vi "Main_Processing.vi"(8 "error in":errorcluster, 11 "Queues in":T1) -> (0 "error out":errorcluster)   [LabVIEW 2019]
uses:
  Queue/TypeDef/#TypeDef_MyRIO_Queues.ctl
  TypeDef/#TypeDef_PropFromDAtoDP.ctl
  Communication/TypeDef/#TypeDef_FromPCtoMR.ctl
  Communication/TypeDef/#TypeDef_Command.ctl
  Communication/TypeDef/#TypeDef_ErrorHandler_prop.ctl
  Communication/TypeDef/#TypeDef_FromMRtoPC.ctl
  Communication/TypeDef/#TypeDef_PropGraph.ctl
  Communication/TypeDef/#TypeDef_PropertiesToSave.ctl
  TypeDef/#TypeDef_EnumOp_DataProcessing.ctl
  Communication/TypeDef/#TypeDef_SetGet.ctl
  TypeDef/#TypeDef_MomentValues.ctl
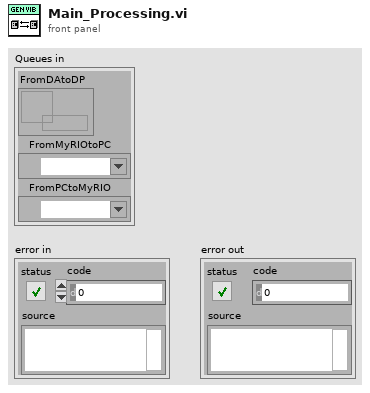
[diagram p1: front panel]
types:
  T1 = typedef "#TypeDef_MyRIO_Queues.ctl" = cluster{"FromDAtoDP":refnum<queue>, "FromMyRIOtoPC":refnum<k21>, "FromPCtoMyRIO":refnum<k21>}
  T2 = typedef "#TypeDef_PropFromDAtoDP.ctl" = cluster{"Accessibility":T3, "RawData":dbl[][], "Counter":i32, "Fs":dbl}
  T3 = typedef "#TypeDef_FromPCtoMR.ctl" = cluster{"Command":T4, "Error?":bool, "Stop":bool, "StopPomiar":bool, "Name":string, "FilesPath":path, "ErrorHandler":T5, "Fs":dbl}
  T4 = typedef "#TypeDef_Command.ctl" = enum16{"Start", "End"}
  T5 = typedef "#TypeDef_ErrorHandler_prop.ctl" = cluster{"Threads":enum16{"Acquisistion", "Data Operation", "Save File"}, "ClearError":bool, "Error Out ":errorcluster, "Error":bool}
  T6 = typedef "#TypeDef_EnumOp_DataProcessing.ctl" = enum16{"Idle", "Init", "Operations", "End", "Error_Shutdown", "ClearError"}
  T7 = typedef "#TypeDef_SetGet.ctl" = enum16{"Set", "Get"}
  T8 = typedef "#TypeDef_MomentValues.ctl" = cluster{"Max":dbl[], "Min":dbl[], "RMS":dbl[], "Init?":bool}
  T9 = typedef "#TypeDef_FromMRtoPC.ctl" = cluster{"Accessibility":T3, "PropGraph":T10, "No Data?":bool, "WaveformData":waveform(dbl)[]}
  T10 = typedef "#TypeDef_PropGraph.ctl" = cluster{"Raw Data":dbl[][], "Poperties":T11, "Power Spectrum / PSD":cluster{"f0":dbl, "df":dbl, "magnitude":dbl[]}[]}
  T11 = typedef "#TypeDef_PropertiesToSave.ctl" = cluster{"RMS values":dbl[], "Max":dbl[], "Min":dbl[], "A(8)":dbl[], "t":dbl, "A(8) Axis":dbl, "Aw":dbl[], "Ak 30min":dbl, "Ak_axis":i32, "Spec":cluster{"f0":dbl, "df":dbl, "magnitude":dbl[]}[]}
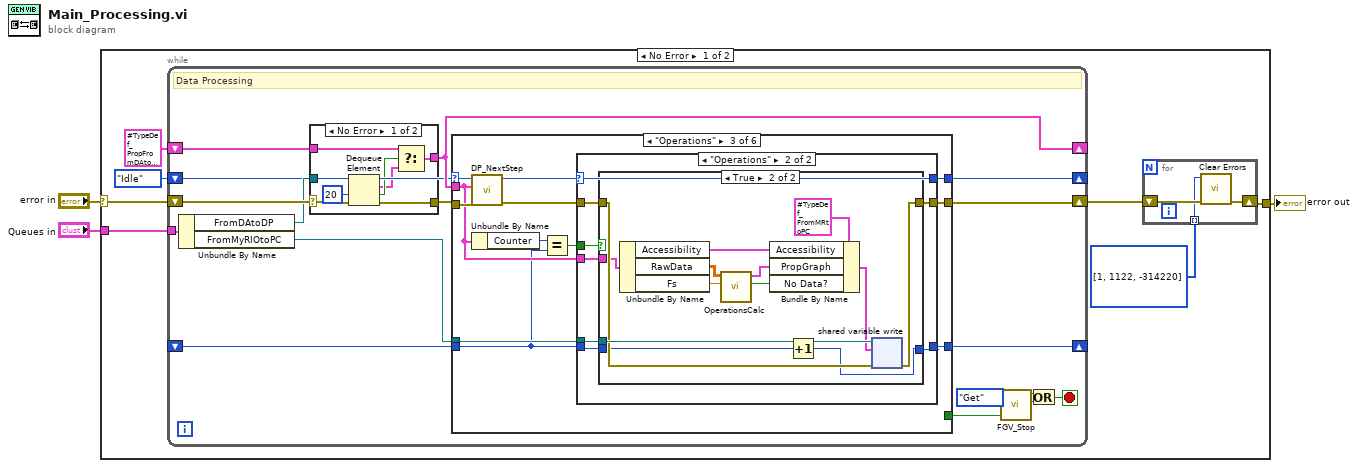
[diagram p0: block diagram]
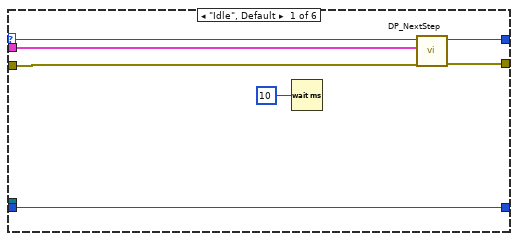
[diagram p3: hidden frame]
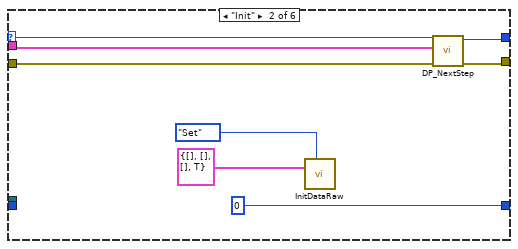
[diagram p4: hidden frame]
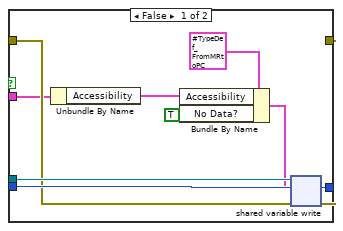
[diagram p6: hidden frame]
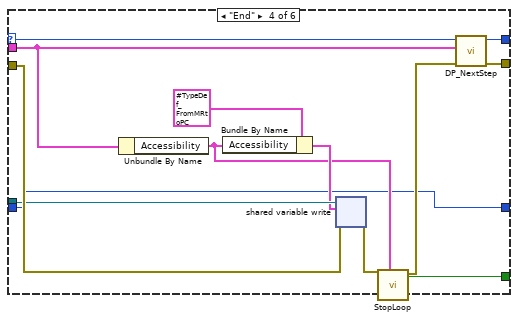
[diagram p7: hidden frame]
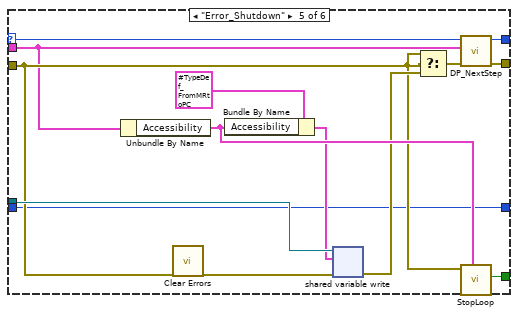
[diagram p8: hidden frame]
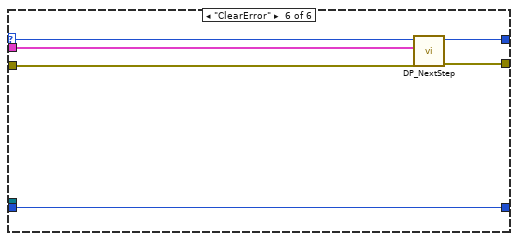
[diagram p9: hidden frame]
diagram:
  n1 = case shown="No Error" "error in" {
    selector: "error in" -> [w10 w133]
    tunnel: "Queues in" -> [w9 _]
    tunnel: [w4 w133] -> w2
    frame No Error {
      n2 = while {
        tunnel: w9 -> [w27]
        shift-right: [w24] -> _
        shift-left: #TypeDef_EnumOp_DataProcessing."Idle" ("EnumOp_DataAcquisition") -> [w21]
        shift-right: [w25] -> w5
        shift-left: w10 -> [w29]
        shift-right: [w22] -> _
        shift-left: T2 {"Accessibility"={"Command"=enum."End", "Error?"=FALSE, "Stop"=FALSE, "StopPomiar"=FALSE, "Name"="", "FilesPath"=path "", "ErrorHandler"={"Threads"=enum."Acquisistion", "ClearError"=FALSE, "Error Out "={"status"=FALSE, "code"=0, "source"=""}, "Error"=FALSE}, "Fs"=0.0}, "RawData"=[], "Counter"=0, "Fs"=0.0} -> [w28]
        shift-right: [w19] -> _
        shift-left: _ -> [w18]
        stop <- w14 stop-if-true
        # "Data Processing"
        n3 = Unbundle By Name(w27) -> ("FromDAtoDP"=w26:refnum<queue>, "FromMyRIOtoPC"=w23:refnum<k21>)
        n4 = case shown="No Error" w29 {
          selector: w29 -> [w34 w39]
          tunnel: [w35 w39] -> w20
          tunnel: [w31 w38] -> w22
          tunnel: w28 -> [w33 w38]
          tunnel: w26 -> [w30 _]
          frame No Error {
            n5 = Dequeue Element(queue=w30, timeout in ms (-1)=20, error in (no error)=w34) -> (element=w32:T2, timed out?=w37:bool, error out=w35:errorcluster)  [unwired: 1 out]
            n6 = Select(t=w33, s=w37, f=w32) -> (s? t:f=w31:T2)
          }
          frame Error {
          }
        }
        n7 = case shown="\"Operations\"" w21 {
          selector: w21 -> [w46 w51 w66 w110 w124 w130]
          tunnel: w20 -> [w42 w54 w64 w108 w115 w128]
          tunnel: w22 -> [w43 w50 w59 w109 w114 w129]
          tunnel: [w45 w53 w63 w112 w126 w132] -> w25
          tunnel: [w44 w52 w60 w111 w125 w131] -> w24
          tunnel: w23 -> [_ _ w65 w107 w122 _]
          tunnel: [_ _ _ w101 w121 _] -> w15
          tunnel: [w40 0 w58 w100 w113 w127] -> w19
          tunnel: w18 -> [w40 _ w57 w100 w113 w127]
          frame "Idle", Default {
            n8 = Wait (ms)(milliseconds to wait=u32 10) -> ()  [unwired: 1 out]
            n9 = call "DP_NextStep.vi"("error in (no error)"=w42, "DAtoDP"=w43, "PreviousStep"=w46) -> ("error out"=w45:errorcluster, "NextStep"=w44:T6)  [unwired: 7 in]
          }
          frame "Init" {
            n10 = call "InitDataRaw.vi"("Get/Set"=#TypeDef_SetGet."Set", "MomentValues in"=T8 {"Max"=[], "Min"=[], "RMS"=[], "Init?"=TRUE}) -> ()  [unwired: 9 in, 1 out]
            n11 = call "DP_NextStep.vi"("error in (no error)"=w54, "DAtoDP"=w50, "PreviousStep"=w51) -> ("error out"=w53:errorcluster, "NextStep"=w52:T6)  [unwired: 7 in]
          }
          frame "Operations" {
            n12 = call "DP_NextStep.vi"("error in (no error)"=w64, "DAtoDP"=w59, "PreviousStep"=w66) -> ("error out"=w62:errorcluster, "NextStep"=w61:T6)  [unwired: 7 in]
            n13 = Unbundle By Name(w59) -> ("Counter"=w56:i32)
            n14 = Equal?(x=w56, y=w57) -> (x = y?=w55:bool)
            n15 = case shown="\"Operations\"" w61 {
              selector: w61 -> [w68 w73]
              tunnel: w65 -> [_ w77]
              tunnel: [w69 w76] -> w63
              tunnel: w62 -> [w69 w75]
              tunnel: w59 -> [_ w74]
              tunnel: [w68 w73] -> w60
              tunnel: w57 -> [w67 w72]
              tunnel: [w67 w71] -> w58
              tunnel: w55 -> [_ w70]
              frame "End", Default {
              }
              frame "Operations" {
                n16 = case shown="True" w70 {
                  tunnel: w77 -> [w85 w98]
                  tunnel: [w83 w93] -> w76
                  tunnel: w75 -> [w84 w92]
                  tunnel: w74 -> [w79 w91]
                  tunnel: w72 -> [w86 w89]
                  tunnel: [w86 w88] -> w71
                  frame False {
                    n17 = Unbundle By Name(w79) -> ("Accessibility"=w78:T3)
                    n18 = Bundle By Name(cluster=T9 {"Accessibility"={"Command"=enum."End", "Error?"=FALSE, "Stop"=FALSE, "StopPomiar"=FALSE, "Name"="", "FilesPath"=path "", "ErrorHandler"={"Threads"=enum."Acquisistion", "ClearError"=FALSE, "Error Out "={"status"=FALSE, "code"=0, "source"=""}, "Error"=FALSE}, "Fs"=0.0}, "PropGraph"={"Raw Data"=[], "Poperties"={"RMS values"=[], "Max"=[], "Min"=[], "A(8)"=[], "t"=0.0, "A(8) Axis"=0.0, "Aw"=[], "Ak 30min"=0.0, "Ak_axis"=0, "Spec"=[]}, "Power Spectrum / PSD"=[]}, "No Data?"=FALSE, "WaveformData"=[]} ("FromMyRiOtoUI"), "Accessibility"=w78, "No Data?"=TRUE) -> (w81:T9)
                    n19 = shared-variable-write(w85, w84, w81) -> (w83:errorcluster)  [unwired: 1 in, 2 out]
                  }
                  frame True {
                    n20 = Unbundle By Name(w91) -> ("Accessibility"=w99:T3, "RawData"=w95:dbl[][], "Fs"=w87:dbl)
                    n21 = call "OperationsCalc.vi"("Fs"=w87, "RawData"=w95) -> ("No Data?"=w90:bool, "PropGraph"=w94:T10)  [unwired: 8 in]
                    n22 = Bundle By Name(cluster=T9 {"Accessibility"={"Command"=enum."End", "Error?"=FALSE, "Stop"=FALSE, "StopPomiar"=FALSE, "Name"="", "FilesPath"=path "", "ErrorHandler"={"Threads"=enum."Acquisistion", "ClearError"=FALSE, "Error Out "={"status"=FALSE, "code"=0, "source"=""}, "Error"=FALSE}, "Fs"=0.0}, "PropGraph"={"Raw Data"=[], "Poperties"={"RMS values"=[], "Max"=[], "Min"=[], "A(8)"=[], "t"=0.0, "A(8) Axis"=0.0, "Aw"=[], "Ak 30min"=0.0, "Ak_axis"=0, "Spec"=[]}, "Power Spectrum / PSD"=[]}, "No Data?"=FALSE, "WaveformData"=[]} ("FromMyRiOtoUI"), "Accessibility"=w99, "PropGraph"=w94, "No Data?"=w90) -> (w97:T9)
                    n23 = Increment(x=w89) -> (x+1=w88:i32)
                    n24 = shared-variable-write(w98, w92, w97) -> (w93:errorcluster)  [unwired: 1 in, 2 out]
                  }
                }
              }
            }
          }
          frame "End" {
            n25 = Unbundle By Name(w109) -> ("Accessibility"=w103:T3)
            n26 = Bundle By Name(cluster=T9 {"Accessibility"={"Command"=enum."End", "Error?"=FALSE, "Stop"=FALSE, "StopPomiar"=FALSE, "Name"="", "FilesPath"=path "", "ErrorHandler"={"Threads"=enum."Acquisistion", "ClearError"=FALSE, "Error Out "={"status"=FALSE, "code"=0, "source"=""}, "Error"=FALSE}, "Fs"=0.0}, "PropGraph"={"Raw Data"=[], "Poperties"={"RMS values"=[], "Max"=[], "Min"=[], "A(8)"=[], "t"=0.0, "A(8) Axis"=0.0, "Aw"=[], "Ak 30min"=0.0, "Ak_axis"=0, "Spec"=[]}, "Power Spectrum / PSD"=[]}, "No Data?"=FALSE, "WaveformData"=[]} ("FromMyRiOtoUI"), "Accessibility"=w103) -> (w105:T9)
            n27 = shared-variable-write(w107, w108, w105) -> (w104:errorcluster)  [unwired: 1 in, 2 out]
            n28 = call "StopLoop.vi"("Accessibility"=w103, "error in (no error)"=w104) -> ("Stop?"=w101:bool, "error out"=w102:errorcluster)  [unwired: 8 in]
            n29 = call "DP_NextStep.vi"("error in (no error)"=w102, "DAtoDP"=w109, "PreviousStep"=w110) -> ("error out"=w112:errorcluster, "NextStep"=w111:T6)  [unwired: 7 in]
          }
          frame "Error_Shutdown" {
            n30 = Unbundle By Name(w114) -> ("Accessibility"=w120:T3)
            n31 = call <vilib>:"Clear Errors.vi"("error in (no error)"=w115) -> ("error out"=w118:errorcluster)  [unwired: 5 in, 1 out]
            n32 = Bundle By Name(cluster=T9 {"Accessibility"={"Command"=enum."End", "Error?"=FALSE, "Stop"=FALSE, "StopPomiar"=FALSE, "Name"="", "FilesPath"=path "", "ErrorHandler"={"Threads"=enum."Acquisistion", "ClearError"=FALSE, "Error Out "={"status"=FALSE, "code"=0, "source"=""}, "Error"=FALSE}, "Fs"=0.0}, "PropGraph"={"Raw Data"=[], "Poperties"={"RMS values"=[], "Max"=[], "Min"=[], "A(8)"=[], "t"=0.0, "A(8) Axis"=0.0, "Aw"=[], "Ak 30min"=0.0, "Ak_axis"=0, "Spec"=[]}, "Power Spectrum / PSD"=[]}, "No Data?"=FALSE, "WaveformData"=[]} ("FromMyRiOtoUI"), "Accessibility"=w120) -> (w119:T9)
            n33 = shared-variable-write(w122, w118, w119) -> (w116:errorcluster)  [unwired: 1 in, 2 out]
            n34 = Select(t=w115, s=w115, f=w116) -> (s? t:f=w117:errorcluster)
            n35 = call "DP_NextStep.vi"("error in (no error)"=w117, "DAtoDP"=w114, "PreviousStep"=w124) -> ("error out"=w126:errorcluster, "NextStep"=w125:T6)  [unwired: 7 in]
            n36 = call "StopLoop.vi"("Accessibility"=w120, "error in (no error)"=w115) -> ("Stop?"=w121:bool)  [unwired: 8 in, 1 out]
          }
          frame "ClearError" {
            n37 = call "DP_NextStep.vi"("error in (no error)"=w128, "DAtoDP"=w129, "PreviousStep"=w130) -> ("error out"=w132:errorcluster, "NextStep"=w131:T6)  [unwired: 7 in]
          }
        }
        n38 = call "FGV_Stop.vi"("Get/Set"=#TypeDef_SetGet."Get") -> ("STOP out"=w16:bool)  [unwired: 10 in]
        n39 = Or(x=w16, y=w15) -> (x .or. y?=w14:bool)
      }
      n40 = for {
        shift-right: [w12] -> w4
        shift-left: w5 -> [w13]
        tunnel: i32[] [1, 1122, -314220] -> [w11] mode=indexing
        n41 = call <vilib>:"Clear Errors.vi"("error in (no error)"=w13, "specific error code to clear (0: all)"=w11) -> ("error out"=w12:errorcluster)  [unwired: 4 in, 1 out]
      }
    }
    frame Error {
    }
  }
  "error out" <- w2
